vi "Create Parameters.vi"(5 "AutoKey":string, 7 "RequestedFields":string[](array[string]), 8 "error in (no error)":errorcluster, 9 "ParameterValues":variant[](array[variant]), 10 "ParameterNames":string[](array[string]), 11 "SqlMapper in":refnum<class "SqlMapper.lvclass">) -> (0 "error out":errorcluster, 2 "Parameters":refnum<class "DynamicParameters.lvclass">, 3 "SqlMapper out":refnum<class "SqlMapper.lvclass">, 4 "FieldNames":string[](array[string]), 6 "ParameterNames Used":string[](array[string]))   [LabVIEW 2020, in "ORM_API.lvlib"]
uses:
  ORM_API.lvlib
  <vilib>/Viviota/shared/ORM.lvlibp/ORM/SqlMapper/SqlMapper.lvclass
  <vilib>/Viviota/shared/ORM.lvlibp/ORM/DynamicParameters/DynamicParameters.lvclass
  <vilib>/Viviota/shared/ORM.lvlibp/ORM/TypeMap/TypeMap.lvclass
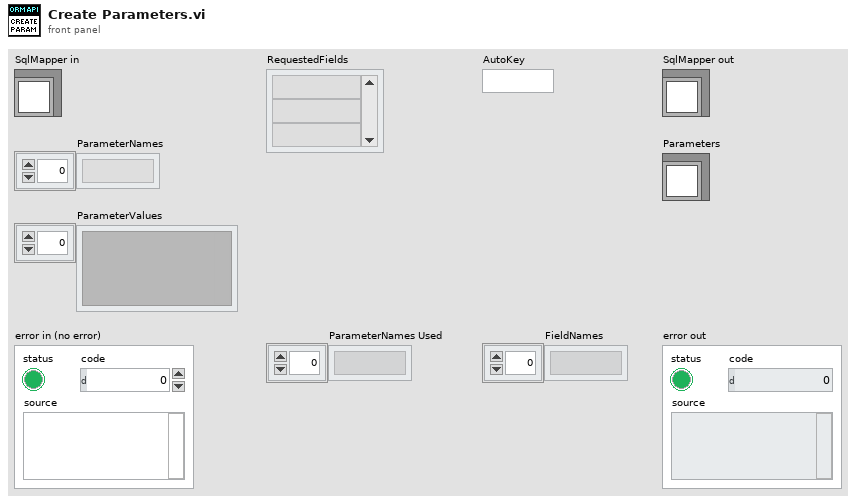
[diagram p1: front panel]
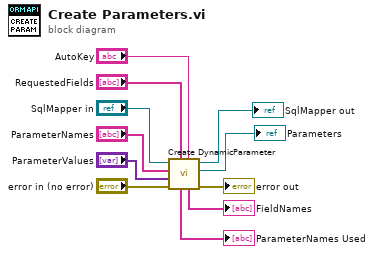
[diagram p0: block diagram]
diagram:
  n1 = call <vilib>:"Create DynamicParameter.vi"("AutoKey"="AutoKey", "RequestedFields"="RequestedFields", "error in (no error)"="error in (no error)", "ParameterValues"="ParameterValues", "ParameterNames"="ParameterNames", "SqlMapper in"="SqlMapper in") -> ("error out"=→"error out":errorcluster, "Parameters"=→"Parameters":refnum<class "DynamicParameters.lvclass">, "SqlMapper out"=→"SqlMapper out":refnum<class "SqlMapper.lvclass">, "FieldNames"=→"FieldNames":string[], "ParameterNames"=→"ParameterNames Used":string[])  [unwired: 1 in]
